vi "Convert Source VI to Resource Data.vi"(8 "error in (no error)":errorcluster, 10 "Use VTT?":bool, 11 "Source VI Ref":refnum<vi>) -> (0 "error out":errorcluster, 1 "BD Resource Data":string, 2 "FP Resource Data":string, 3 "Resources":T1)   [LabVIEW 2023]
uses:
  Resource Manipulation.lvlib
  Resource Manipulation/Find Resource by Type (String).vi
  Resource Manipulation/Resource.ctl
  Resource Manipulation/Resource Array.ctl
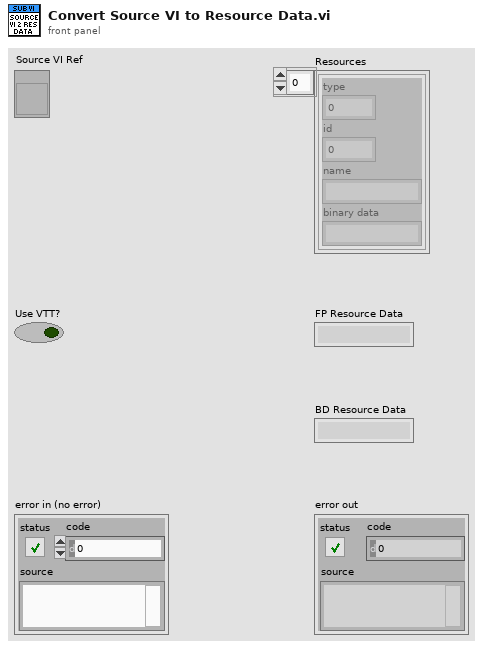
[diagram p1: front panel]
types:
  T1 = typedef "Resource Manipulation.lvlib/Resource Array.ctl" = T2[]
  T2 = typedef "Resource Manipulation.lvlib/Resource.ctl" = cluster{"type":u32, "id":i32, "name":string, "binary data":string}
  T3 = typedef "Resource Manipulation.lvlib/Heap Save Format.ctl" = u16
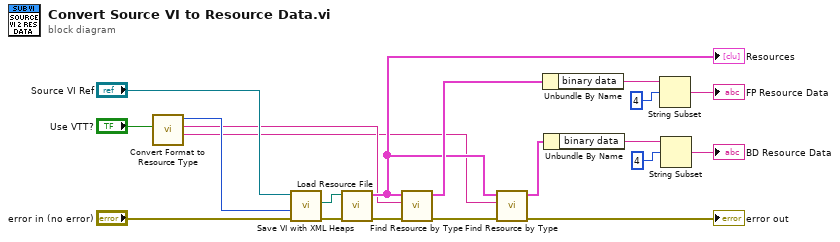
[diagram p0: block diagram]
diagram:
  n1 = call "Convert Format to Resource Type.vi"("Use VTT?"="Use VTT?") -> ("BD Resource Type"=w3:string, "FP Resource Type"=w4:string, "Heap Save Format"=w10:T3)  [unwired: 8 in]
  n2 = call "Save VI with XML Heaps.vi"("error in (no error)"="error in (no error)", "Heap Save Format (1=XML)"=w10, "VI Refnum In"="Source VI Ref") -> ("error out"=w13:errorcluster, "VI Path out"=w20:path)  [unwired: 6 in, 1 out]
  n3 = call "Load Resource File.vi"("error in (no error)"=w13, "Resource File"=w20) -> ("error out"=w9:errorcluster, "Resources"=w5:T1)  [unwired: 7 in, 1 out]
  "Resources" <- w5
  n4 = call-poly "Find Resource by Type.vi"("error in (no error)"=w9, "Resource Type"=w4, "Resources"=w5) -> ("error out"=w8:errorcluster, "Resource"=w17:T2)  [unwired: 5 in, 2 out]
  n5 = call-poly "Find Resource by Type.vi"("error in (no error)"=w8, "Resource Type"=w3, "Resources"=w5) -> ("error out"=→"error out":errorcluster, "Resource"=w14:T2)  [unwired: 5 in, 2 out]
  n6 = Unbundle By Name(w17) -> ("binary data"=w19:string)
  n7 = Unbundle By Name(w14) -> ("binary data"=w15:string)
  n8 = String Subset(string=w19, offset (0)=4) -> (substring=→"FP Resource Data":string)  [unwired: 1 in]
  n9 = String Subset(string=w15, offset (0)=4) -> (substring=→"BD Resource Data":string)  [unwired: 1 in]
